vi "Initialise Text.vi"(8 "error in (no error)":errorcluster, 10 "Renderer":u32, 11 "Ship in":refnum<class "Ship.lvclass">) -> (0 "error out":errorcluster, 3 "Ship out":refnum<class "Ship.lvclass">)   [LabVIEW 2021, in "Ship.lvclass"]
uses:
  Ship.lvclass
  Ship.lvclass/Ship.ctl
  <vilib>/numeric/Random Number (Range) I64.vi
  <vilib>/numeric/sub_Random U32.vi
  <vilib>/Utility/file.llb/Application Directory.vi
  Resource Manager/Resource Manager.lvclass
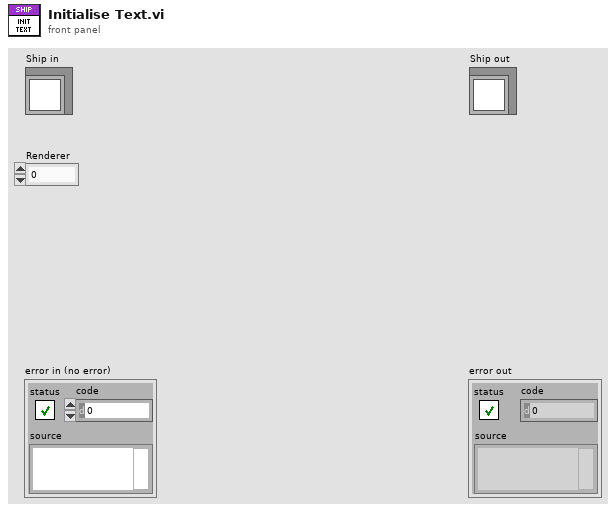
[diagram p1: front panel]
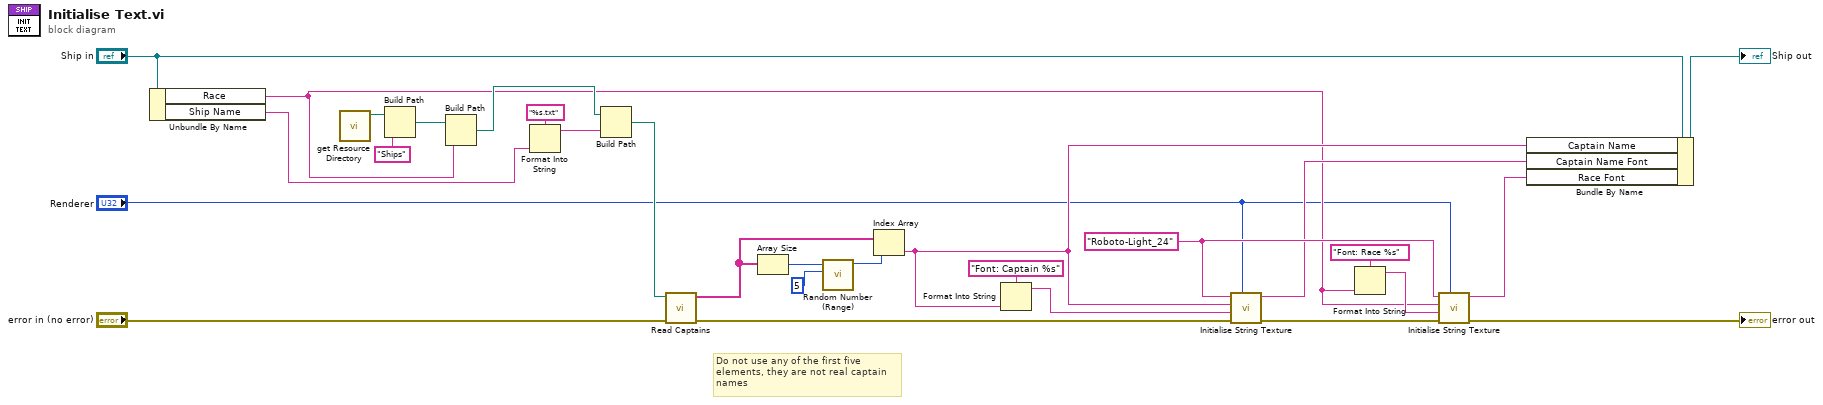
[diagram p0: block diagram]
diagram:
  w19 = "Roboto-Light_24" ("Font Combo")
  # "Do not use any of the first five elements, they are not real captain names"
  n1 = Unbundle By Name("Ship in") -> ("Race"=w7:string, "Ship Name"=w22:string)
  n2 = call "get Resource Directory.vi"() -> ("Resource Directory"=w26:path)  [unwired: 11 in]
  n3 = Build Path(base path=w26, name or relative path="Ships") -> (appended path=w28:path)
  n4 = Build Path(base path=w28, name or relative path=w7) -> (appended path=w23:path)
  n5 = Format Into String(format string="%s.txt", w22) -> (resulting string=w25:string)  [unwired: 2 in, 1 out]
  n6 = Build Path(base path=w23, name or relative path=w25) -> (appended path=w12:path)
  n7 = call "Read Captains.vi"("error in (no error)"="error in (no error)", "Captains"=w12) -> ("error out"=w15:errorcluster, "Captains"=w14:string[])  [unwired: 8 in]
  n8 = Array Size(array=w14) -> (size(s)=w3:i32)
  n9 = call-poly <vilib>:"Random Number (Range).vi"("lower bound (-100)"=5 ("Low"), "upper bound (100)"=w3) -> ("number"=w1:i64)  [unwired: 9 in]
  n10 = Index Array(array=w14, index=w1) -> (element=w10:string)
  n11 = Format Into String(format string="Font: Captain %s", w10) -> (resulting string=w17:string)  [unwired: 2 in, 1 out]
  n12 = call "Initialise String Texture.vi"("Renderer"="Renderer", "error in (no error)"=w15, "Name"=w17, "Text"=w10, "Font Combo"=w19) -> ("error out"=w18:errorcluster, "Name In Cache"=w9:string)  [unwired: 5 in]
  n13 = Format Into String(format string="Font: Race %s", w7) -> (resulting string=w21:string)  [unwired: 2 in, 1 out]
  n14 = call "Initialise String Texture.vi"("Renderer"="Renderer", "error in (no error)"=w18, "Name"=w21, "Text"=w7, "Font Combo"=w19) -> ("error out"=→"error out":errorcluster, "Name In Cache"=w8:string)  [unwired: 5 in]
  n15 = Bundle By Name(cluster="Ship in", "Captain Name"=w10, "Captain Name Font"=w9, "Race Font"=w8) -> (→"Ship out":refnum<class "Ship.lvclass">)
